vi "Find 2nd_Spike after a large one.vi"(6 "Spikes Array In":cluster{"Index":i32, "max value":dbl}[](array[cluster]), 7 "Block Mean":dbl, 9 "Number of samples":i32, 10 "Time Trace in":dbl[](array[numeric]), 11 "Cut Value":dbl) -> (2 "Time Trace out":dbl[](array[numeric]), 4 "Spikes Array Out":cluster{"Index":i32, "max value":dbl}[](array[cluster]))   [LabVIEW 2018]
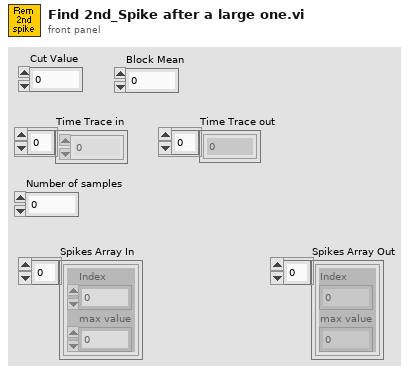
[diagram p1: front panel]
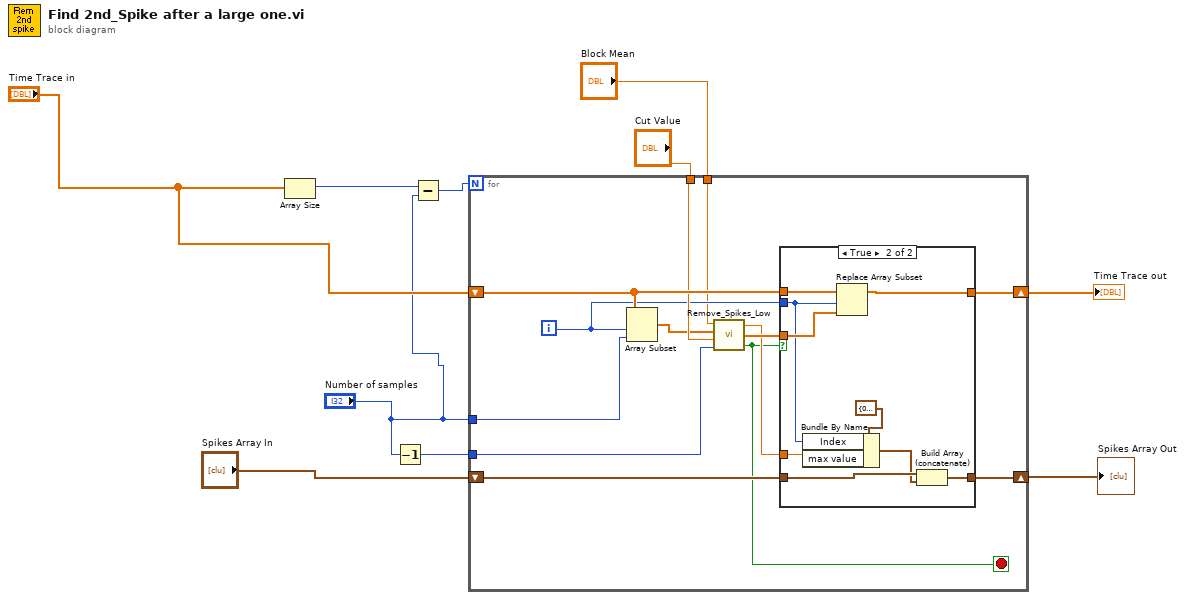
[diagram p0: block diagram]
diagram:
  n1 = Array Size(array="Time Trace in") -> (size(s)=w5:i32)
  n2 = Decrement(x="Number of samples") -> (x-1=w7:i32)
  n3 = Subtract(x=w5, y="Number of samples") -> (x-y=w3:i32)
  n4 = for {
    N: w3 -> [_]
    shift-right: [w20] -> w10
    shift-left: "Time Trace in" -> [w21]
    tunnel: "Number of samples" -> [w23]
    tunnel: w7 -> [w22]
    tunnel: "Cut Value" -> [w19]
    shift-right: [w18] -> w9
    shift-left: "Spikes Array In" -> [w17]
    tunnel: "Block Mean" -> [w11]
    i -> [w13]
    stop <- w12 stop-if-true
    n5 = Array Subset(array=w21, index=w13, length=w23) -> (w15:dbl[])
    n6 = call "Remove_Spikes_Low.vi"("index"=w22, "Background noise"=w19, "Time Trace"=w15, "Block Mean"=w11) -> ("Spike"=w12:bool, "Filtered Time Trace"=w16:dbl[], "max value"=w14:dbl)
    n7 = case shown="True" w12 {
      tunnel: w13 -> [_ w31]
      tunnel: w16 -> [_ w34]
      tunnel: w21 -> [w25 w33]
      tunnel: [w25 w32] -> w20
      tunnel: [w24 w28] -> w18
      tunnel: w17 -> [w24 w29]
      tunnel: w14 -> [_ w30]
      frame False {
      }
      frame True {
        n8 = Bundle By Name(cluster=cluster{"Index":i32, "max value":dbl} {"Index"=0, "max value"=0.0} ("output cluster"), "Index"=w31, "max value"=w30) -> (w27:cluster{"Index":i32, "max value":dbl})
        n9 = Replace Array Subset(array=w33, new element=w34, index=w31) -> (w32:dbl[])
        n10 = Build Array (concatenate)(w29, w27) -> (w28:cluster{"Index":i32, "max value":dbl}[])
      }
    }
  }
  "Time Trace out" <- w10
  "Spikes Array Out" <- w9
